vi "Reset Min and Max.vi"(8 "error in (no error)":errorcluster, 11 "VISA resource name":refnum<visa-resource-name>) -> (0 "error out":errorcluster, 3 "VISA resource name out":refnum<visa-resource-name>)   [LabVIEW 2015, in "Lake Shore 350.lvlib"]
doc: "Resets the Min/Max data function. Minimum and maximum data for all inputs in reset."
uses:
  Lake Shore 350.lvlib
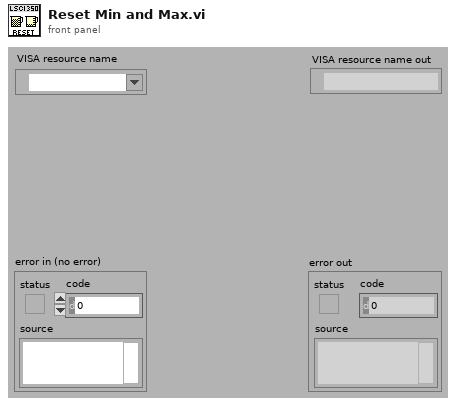
[diagram p1: front panel]
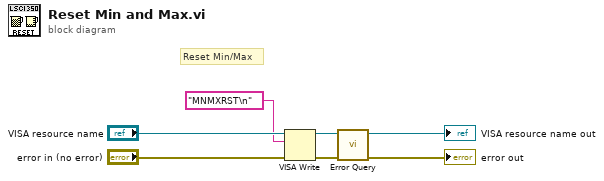
[diagram p0: block diagram]
diagram:
  # "Reset Min/Max"
  n1 = VISA Write(VISA resource name="VISA resource name", write buffer="MNMXRST\n", error in (no error)="error in (no error)") -> (VISA resource name out=w2:refnum<visa-resource-name>, error out=w3:errorcluster)  [unwired: 1 out]
  n2 = call "Error Query.vi"("error in (no error)"=w3, "VISA resource name"=w2) -> ("error out"=→"error out":errorcluster, "VISA resource name out"=→"VISA resource name out":refnum<visa-resource-name>)  [unwired: 7 in, 1 out]
